vi "PCO_GetCoolingSetpointTemperature.vi"(8 "error in (no error)":errorcluster {"code" format="%x"}, 11 "ph":u64) -> (0 "error out":errorcluster {"code" format="%x"}, 1 "sCoolSet":i16, 2 "ErrorMessage":i32 format="%x", 3 "ph out":u64)   [LabVIEW 2019, in "SDK.lvlib" / "ImageSensor.lvlib"]
doc: "<b>Description:</b>\nThis function returns the temperature setpoint for the image sensor.\nThe current sensor temperature can be read out with the PCO_GetTemperature function.\n\n<b>Supported camera type:</b>\nAll cameras\n\n<b>Descriptor dependency:</b>\ndwGeneralCapsDESC1: COOLING_SETPOINTS"
uses:
  ImageSensor.lvlib
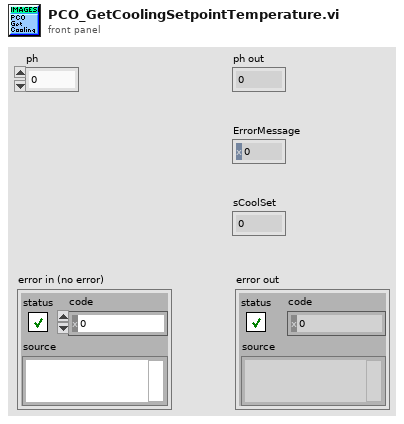
[diagram p1: front panel]
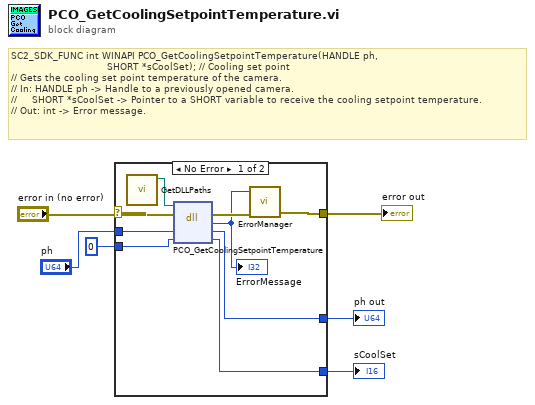
[diagram p0: block diagram]
diagram:
  # "SC2_SDK_FUNC int WINAPI PCO_GetCoolingSetpointTemperature(HANDLE ph,\n                                SHORT *sCoolSet); // Cooling set point\n// Gets the cooling set point temperature of the camera.\n// In: HANDLE ph -> Handle to a previously opened camera.\n//     SHORT *sCoolSet -> Pointer to a SHORT variable to receive the cooling setpoint temperature.\n// Out: int -> Error message."
  n1 = case shown="No Error" "error in (no error)" {
    selector: "error in (no error)" -> [w8 w18]
    tunnel: "ph" -> [w15 w17]
    tunnel: i16 0 ("sCoolSet") -> [w14 w16]
    tunnel: [w13 w16] -> w4
    tunnel: [w12 w17] -> w3
    tunnel: [w11 w18] -> w2
    frame No Error {
      n2 = call "GetDLLPaths.vi"() -> ("SC2_Cam_Path"=w7:path)  [unwired: 9 in, 2 out]
      n3 = dll-call lib="?" fn="PCO_GetCoolingSetpointTemperature"(path in=w7, error in=w8, "ph"=w15, "sCoolSet"=w14) -> (error out=w10:errorcluster, "return type"=w9:i32, "ph"=w12:u64, "sCoolSet"=w13:i16)  [unwired: 1 in, 1 out]
      "ErrorMessage" <- w9
      n4 = call "ErrorManager.vi"("error in (no error)"=w10, "error code"=w9) -> ("error out"=w11:errorcluster)  [unwired: 3 in]
    }
    frame Error {
    }
  }
  "ph out" <- w3
  "sCoolSet" <- w4
  "error out" <- w2
